vi "practica1_1.2.vi"() -> ()   [LabVIEW 2016]
panel:
  in  "String":string
  out "String":string
  out "Thermometer":dbl(slide) scale=0.0..100.0
  in  "DBL":dbl(knob) scale=0.0..100.0
  out "boleano":bool
  out "INT":i32
  in  "INT":i32
  in  "boleano":bool
  # "en este solo se muestran dos estados\nTRUE o FALSE los cual se muestra por \nla luz encendida o apagada"
  # "en este se muestran unicamente\nnuemeros enteros"
  # "en este se pueden ver todos los numeros \nya sean flotantes o enteros en un rango\nque aparece en el knop"
  # "en este se muestran las palabras que se \nponen en el renglon de arriba"
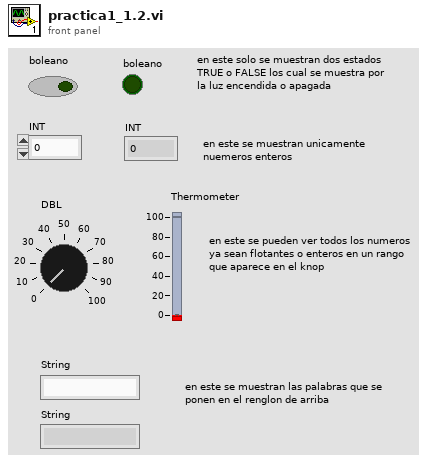
[diagram p1: front panel]
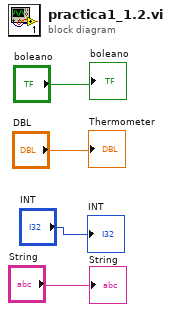
[diagram p0: block diagram]
diagram:
  "INT" <- "INT"
  "boleano" <- "boleano"
  "Thermometer" <- "DBL"
  "String" <- "String"
